vi "Set.vi"(8 "error in (no error)":errorcluster, 10 "Variant":variant, 11 "Ref":refnum<queue>) -> (0 "error out":errorcluster, 3 "Ref out":refnum<queue>)   [LabVIEW 2016, in "SEQ.lvlib"]
doc: "Set the Single Element Queued (SEQ) based variable in variant format."
uses:
  SEQ.lvlib
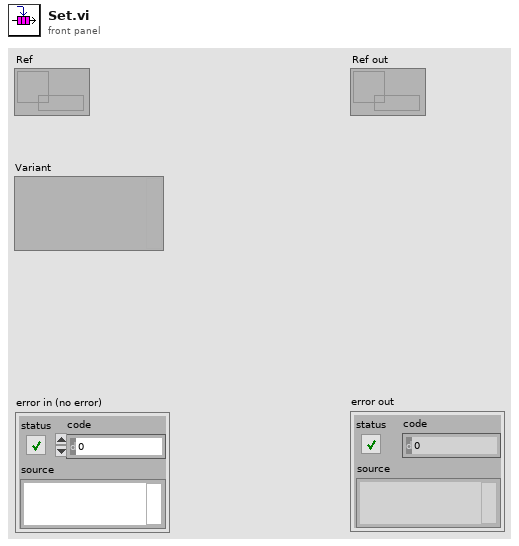
[diagram p1: front panel]
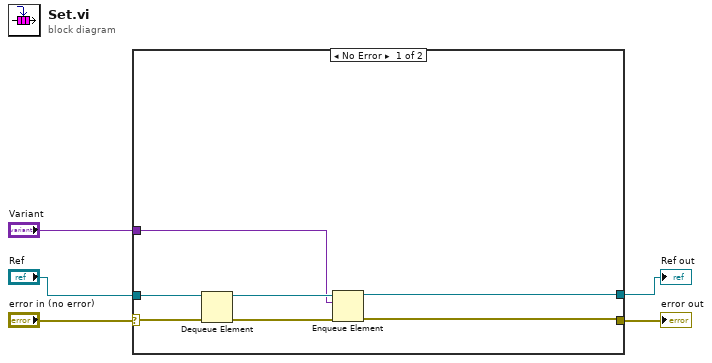
[diagram p0: block diagram]
diagram:
  n1 = case shown="No Error" "error in (no error)" {
    selector: "error in (no error)" -> [w12 w13]
    tunnel: [w9 w13] -> w5
    tunnel: [w8 _] -> w2
    tunnel: "Ref" -> [w7 _]
    tunnel: "Variant" -> [w6 _]
    frame No Error {
      n2 = Dequeue Element(queue=w7, error in (no error)=w12) -> (queue out=w10:refnum<queue>, error out=w11:errorcluster)  [unwired: 1 in, 2 out]
      n3 = Enqueue Element(queue=w10, element=w6, error in (no error)=w11) -> (queue out=w8:refnum<queue>, error out=w9:errorcluster)  [unwired: 1 in, 1 out]
    }
    frame Error {
    }
  }
  "error out" <- w5
  "Ref out" <- w2
